vi "Has Destroyed.vi"(7 "Sender":refnum<class "Sender.lvclass">, 9 "Error":errorcluster, 10 "Actor":refnum<class "Actor.lvclass">, 11 "Base Actor in":refnum<class "Base Actor.lvclass">) -> (0 "Error out":errorcluster, 3 "Base Actor out":refnum<class "Base Actor.lvclass">)   [LabVIEW 2020, in "jettl.lvlib" / "Actor.lvlib" / "Base Actor.lvclass"]
uses:
  Base Actor.lvclass
  Actor/Actor.lvclass
  Sender/Sender/Sender.lvclass
  Base Actor.lvclass/Base Actor.ctl
  Attributes/Attributes/Attributes.lvclass
  Actor.lvlib
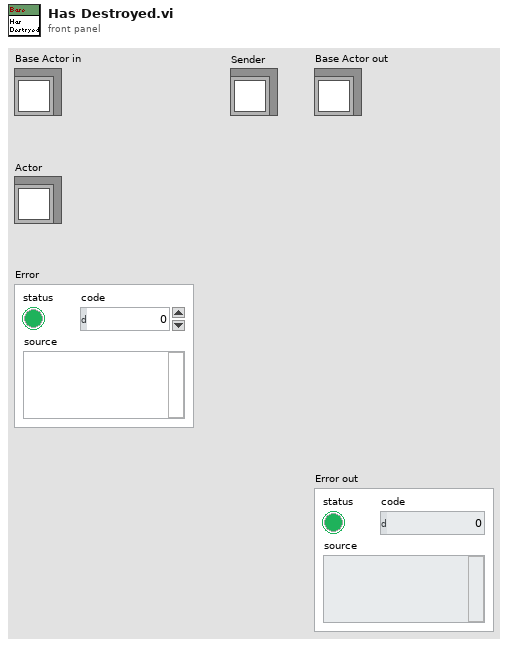
[diagram p1: front panel]
types:
  T1 = typedef "jettl.lvlib/Actor.lvlib/Relation.ctl" = enum16{"Self", "Creator", "Created"}
  T2 = typedef "jettl.lvlib/Actor.lvlib/Created Attributes Map.ctl" = map{string, refnum<class "Attributes.lvclass">}
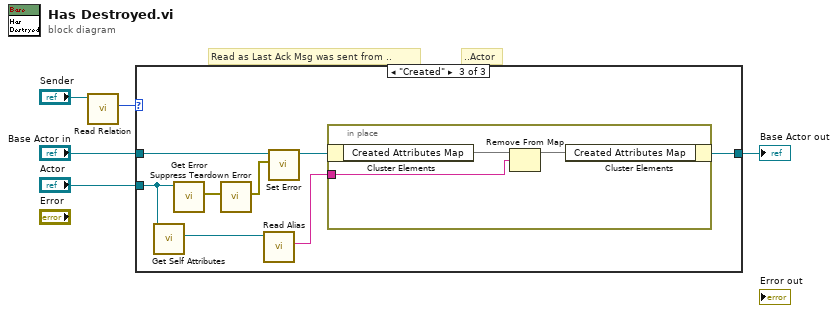
[diagram p0: block diagram]
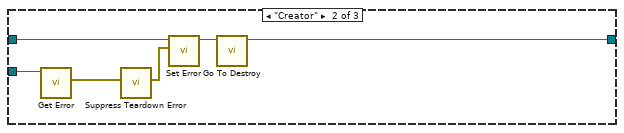
[diagram p3: hidden frame]
diagram:
  # "..Actor"
  # "Read as Last Ack Msg was sent from .."
  n1 = call-dynamic "Read Relation.vi"("Sender in"="Sender") -> ("Relation"=w1:T1)  [unwired: 10 in]
  n2 = case shown="\"Created\"" w1 {
    tunnel: "Base Actor in" -> [w6 w9 w18]
    tunnel: [w6 w12 w13] -> w5
    tunnel: "Actor" -> [_ w11 w20]
    frame "Self" {
      # "Case will not fundamentally execute"
    }
    frame "Creator" {
      n3 = call-dynamic "Get Error.vi"("Actor in"=w11) -> ("Error"=w10:errorcluster)  [unwired: 10 in]
      n4 = call "Suppress Teardown Error.vi"("Error in"=w10) -> ("Error out"=w7:errorcluster)  [unwired: 10 in]
      n5 = call-dynamic "Set Error.vi"("Error"=w7, "Base Actor in"=w9) -> ("Base Actor out"=w8:refnum<class "Base Actor.lvclass">)  [unwired: 9 in]
      n6 = call-dynamic "Go To Destroy.vi"("Base Actor in"=w8) -> ("Base Actor out"=w12:refnum<class "Base Actor.lvclass">)  [unwired: 9 in, 1 out]
    }
    frame "Created" {
      n7 = call-dynamic "Get Self Attributes.vi"("Actor in"=w20) -> ("Self Attributes"=w16:refnum<class "Attributes.lvclass">)  [unwired: 10 in]
      n8 = call-dynamic "Get Error.vi"("Actor in"=w20) -> ("Error"=w19:errorcluster)  [unwired: 10 in]
      n9 = call "Suppress Teardown Error.vi"("Error in"=w19) -> ("Error out"=w17:errorcluster)  [unwired: 10 in]
      n10 = call-dynamic "Read Alias.vi"("Attributes in"=w16) -> ("Alias"=w15:string)  [unwired: 10 in]
      n11 = call-dynamic "Set Error.vi"("Error"=w17, "Base Actor in"=w18) -> ("Base Actor out"=w14:refnum<class "Base Actor.lvclass">)  [unwired: 9 in]
      n12 = in-place {
        in-place-border: w15 -> [w21]
        n13 = in-place-cluster #1(w14) -> ("Created Attributes Map"=w23:T2)
        n14 = Remove From Map(10:w21, 11:w23) -> (3:w22:T2)  [unwired: 2 out]
        n15 = in-place-cluster #1("Created Attributes Map"=w22) -> (w13:refnum<class "Base Actor.lvclass">)
      }
    }
  }
  "Base Actor out" <- w5
